vi "Pulse Measurements N chan.vi"(5 "export mode":u16(ring) items=["all", "no period and duty cycle"], 6 "percent level settings":T3={"method"=enum."auto select", "histogram size"=256, "histogram method"=enum."mode", "reserved"=1.0} {"reserved" format="%0.2f"}, 7 "pulse number (1)":i32=1 min=1, 8 "error in (no error)":errorcluster, 9 "reference levels":T2={"high ref level"=90.0, "mid ref level"=50.0, "low ref level"=10.0, "ref units"=1} {"ref units" items=["absolute", "percent"]; "high ref level" format="%.2p"; "low ref level" format="%.2p"; "mid ref level" format="%.2p"}, 10 "polarity (high)":u16(ring)=1 items=["low pulse", "high pulse"], 11 "signal(s) in":waveform(dbl)[](array[waveform])) -> (0 "error out":errorcluster, 1 "duty cycle":dbl[](array[numeric]) format="%.2p", 2 "pulse duration":dbl[](array[numeric]) format="%.2p", 3 "period":dbl[](array[numeric]) format="%.2p", 4 "measurement info":T1(array[cluster]))   [LabVIEW 2020, in "NI_MAPro.lvlib"]
doc: "Accepts a periodic waveform or an array of periodic waveforms and returns the <B>period</B>, <B>pulse duration</B> (pulse width), <B>duty cycle</B> (duty factor), and <B>pulse center</B> of a selected pulse and period. Wire data to the <B>signal in</B> input to determine the polymorphic instance to use or manually select the instance."
uses:
  NI_MAPro.lvlib
  NI_MABase.lvlib
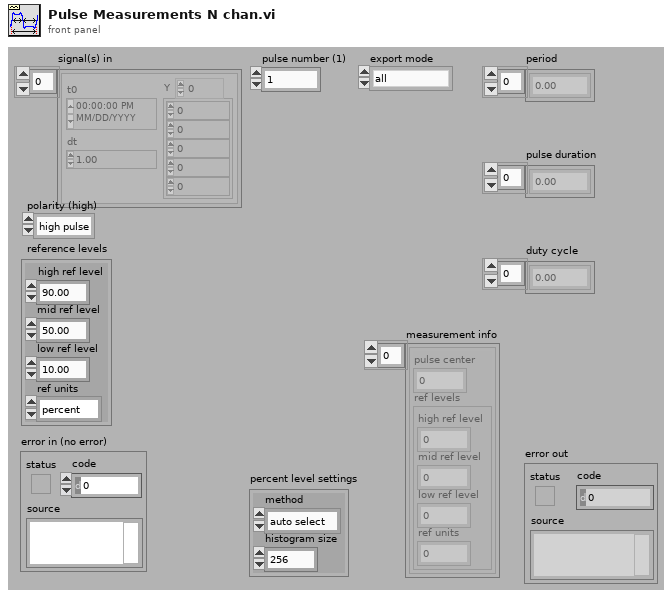
[diagram p1: front panel]
types:
  T1 = cluster{"pulse center":dbl, "ref levels":cluster{"high ref level":dbl, "mid ref level":dbl, "low ref level":dbl, "ref units":u16}}[]
  T2 = cluster{"high ref level":dbl, "mid ref level":dbl, "low ref level":dbl, "ref units":u16}
  T3 = cluster{"method":enum32{"histogram", "peak", "auto select"}, "histogram size":i32, "histogram method":enum16{"mode"}, "reserved":dbl}
  T4 = cluster{"pulse center":dbl, "ref levels":cluster{"high ref level":dbl, "mid ref level":dbl, "low ref level":dbl, "ref units":u16}}
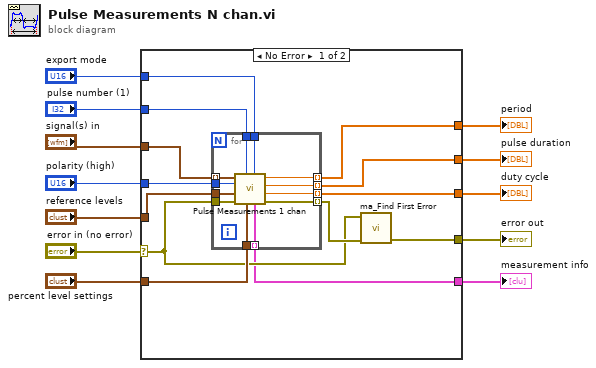
[diagram p0: block diagram]
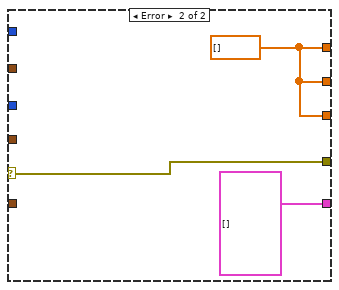
[diagram p2: hidden frame]
diagram:
  n1 = case shown="No Error" "error in (no error)" {
    selector: "error in (no error)" -> [w19 w40]
    tunnel: "percent level settings" -> [w24 _]
    tunnel: [w18 w40] -> w10
    tunnel: "signal(s) in" -> [w25 _]
    tunnel: [w23 w38] -> w8
    tunnel: [w22 w38] -> w7
    tunnel: [w21 w38] -> w6
    tunnel: "reference levels" -> [w17 _]
    tunnel: "pulse number (1)" -> [w16 _]
    tunnel: "polarity (high)" -> [w15 _]
    tunnel: [w14 T1 []] -> w2
    tunnel: "export mode" -> [w13 _]
    frame No Error {
      n2 = for {
        tunnel: w19 -> [w37]
        tunnel: w24 -> [w36]
        tunnel: [w35] -> w20 mode=indexing
        tunnel: [w34] -> w23 mode=indexing
        tunnel: [w33] -> w22 mode=indexing
        tunnel: [w32] -> w21 mode=indexing
        tunnel: w25 -> [w31] mode=indexing
        tunnel: w17 -> [w30]
        tunnel: w16 -> [w29]
        tunnel: w15 -> [w28]
        tunnel: [w27] -> w14 mode=indexing
        tunnel: w13 -> [w26]
        n3 = call "Pulse Measurements 1 chan.vi"("export mode"=w26, "percent level settings"=w36, "pulse number (1)"=w29, "error in (no error)"=w37, "reference levels"=w30, "polarity (high)"=w28, "signal in"=w31) -> ("error out"=w35:errorcluster, "duty cycle"=w32:dbl, "pulse duration"=w33:dbl, "period"=w34:dbl, "measurement info"=w27:T4)
      }
      n4 = call "ma_Find First Error.vi"("error array in"=w20, "error in 1 (no error)"=w19) -> ("error out"=w18:errorcluster)  [unwired: 2 in, 3 out]
    }
    frame Error {
      w38 = dbl[] []
    }
  }
  "error out" <- w10
  "period" <- w8
  "pulse duration" <- w7
  "duty cycle" <- w6
  "measurement info" <- w2
